vi "Usun kursor.vi"(8 "error in (no error)":errorcluster) -> (0 "error out":errorcluster)   [LabVIEW 2013]
doc: "Usuwa kursory\nustawione"
uses:
  <vilib>/Utility/miscctls.llb/LVCursorListTypeDef.ctl
panel:
  in  "All":bool
  in  "Cancel":bool
  in  "OK":bool
  in  "Lista kursorów":i32(listbox)
  in  "Wykres Ref":refnum<vi>
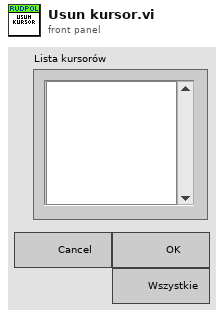
[diagram p1: front panel]
types:
  T1 = typedef "LVCursorListTypeDef.ctl" = cluster{"Name":string, "Color":u32, "Style":u8, "Point Style":u8, "Name Visible":bool, "Allow Drag":bool, "Cursor Mode":u32, "Plot":i32, "Index":i32, "Position":cluster{"X":dbl, "Y":dbl}, "X Scale":u32, "Y Scale":u32, "Watch Plots":i32[], "Watch All Plots":bool, "Plot Area":i32, "Label Offset":cluster{"X":dbl, "Y":dbl}}[]
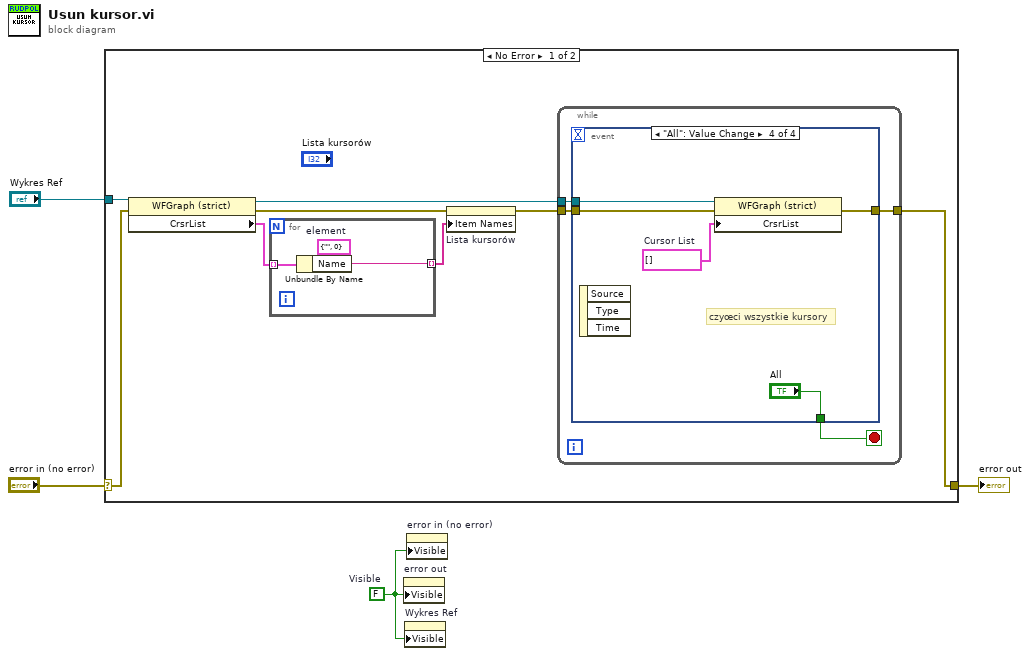
[diagram p0: block diagram]
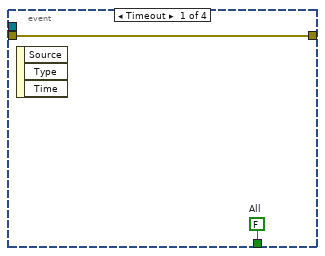
[diagram p2: hidden frame]
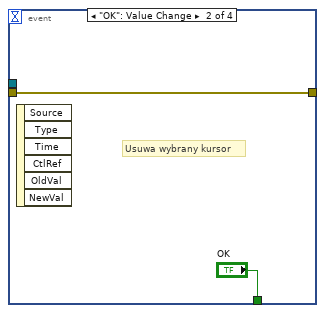
[diagram p3: hidden frame]
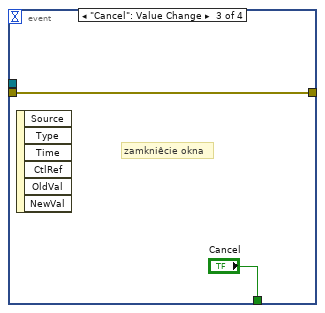
[diagram p4: hidden frame]
diagram:
  w1 = FALSE  # Visible
  n1 = case shown="No Error" "error in (no error)" {
    selector: "error in (no error)" -> [w11 w30]
    tunnel: [w5 w30] -> w3
    tunnel: "Wykres Ref" -> [w12 _]
    frame No Error {
      n2 = property class="WFGraph (strict)"(reference=w12, error in=w11) -> (reference out=w7:refnum<vi>, error out=w8:errorcluster, "CrsrList"=w10:T1)
      n3 = for {
        tunnel: w10 -> [w14] mode=indexing
        tunnel: [w13] -> w9 mode=indexing
        (unwired) cluster{"String":string, "Value":u16} {"String"="", "Value"=0}  # element
        n4 = Unbundle By Name(w14) -> ("Name"=w13:string)
      }
      n5 = property on="Lista kursorów" class="LstBox (strict)"(error in=w8, "Item Names"=w9) -> (error out=w6:errorcluster)  [unwired: 1 in, 1 out]
      n6 = while {
        tunnel: w7 -> [w17]
        tunnel: w6 -> [w16]
        tunnel: [w15] -> w5
        stop <- w18 stop-if-true
        n7 = event shown="[3] \"All\": Value Change" {
          selector: _ -> [_ _ _ _]
          dyn-events: _ -> [_ _ _ _]
          timeout: _ -> [_ _ _ _]
          tunnel: [w19 "OK" "Cancel" "All"] -> w18
          tunnel: w17 -> [_ _ _ w28]
          tunnel: w16 -> [w20 w21 w23 w27]
          tunnel: [w20 w21 w23 w25] -> w15
          event Timeout {
            w19 = FALSE  # All
            n8 = event-data() -> ()  [unwired: 1 in, 3 out]
          }
          event "OK": Value Change {
            # "Usuwa wybrany kursor"
            n9 = event-data() -> ()  [unwired: 1 in, 6 out]
          }
          event "Cancel": Value Change {
            # "zamkniêcie okna"
            n10 = event-data() -> ()  [unwired: 1 in, 6 out]
          }
          event "All": Value Change {
            w26 = T1 []  # Cursor List
            # "czyœci wszystkie kursory"
            n11 = event-data() -> ()  [unwired: 1 in, 3 out]
            n12 = property class="WFGraph (strict)"(reference=w28, error in=w27, "CrsrList"=w26) -> (error out=w25:errorcluster)  [unwired: 1 out]
          }
        }
      }
    }
    frame Error {
    }
  }
  "error out" <- w3
  n13 = property on="error out" class="Clust (strict)"("Visible"=w1) -> ()  [unwired: 2 in, 2 out]
  n14 = property on="Wykres Ref" class="LVObjRef (strict)"("Visible"=w1) -> ()  [unwired: 2 in, 2 out]
  n15 = property on="error in (no error)" class="Clust (strict)"("Visible"=w1) -> ()  [unwired: 2 in, 2 out]
